vi "XYZ Table Stage Module.vi"(7 "Action":T4, 8 "Error In":errorcluster, 10 "Axis":enum16{"X Axis", "Y Axis", "Z Axis"}(ring), 11 "Control Param In":T2={"Position"=0.0, "Is.Enabled?"=FALSE, "Is.Connected?"=FALSE, "Device SN"="45876539", "AccelerationMaximum"=0.0, "VelocityMaximum"=0.0, "Acceleration"=0.0, "Velocity"=0.0, "waitTimeout (ms)"=0, "Model"=enum."None", "Is.Homed?"=FALSE}) -> (0 "Error Out":errorcluster)   [LabVIEW 2014]
uses:
  Controls/Translation Stage Cluster.ctl
  General/Controls/Translation Stage Types.ctl
  Controls/Motion Translation Module Control.ctl
  General/Controls/Set Get Controls.ctl
  HW Configurations.vi
  General/Controls/FGV Actions.ctl
panel:
  in  "Set/Get":T1=enum."Get"
  out "Control Param Out":T2={"Position"=0.0, "Is.Enabled?"=FALSE, "Is.Connected?"=FALSE, "Device SN"="45876539", "AccelerationMaximum"=0.0, "VelocityMaximum"=0.0, "Acceleration"=0.0, "Velocity"=0.0, "waitTimeout (ms)"=0, "Model"=enum."None", "Is.Homed?"=FALSE}
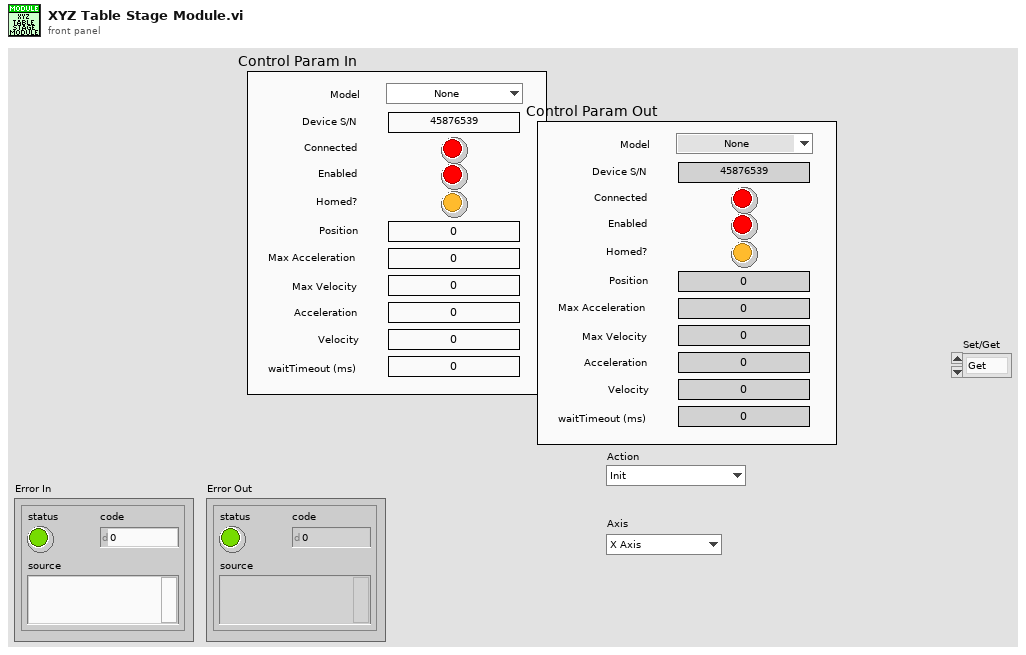
[diagram p1: front panel]
types:
  T1 = typedef "Set Get Controls.ctl" = enum16{"Set", "Get"}
  T2 = typedef "Translation Stage Cluster.ctl" = cluster{"Position":dbl, "Is.Enabled?":bool, "Is.Connected?":bool, "Device SN":string, "AccelerationMaximum":dbl, "VelocityMaximum":dbl, "Acceleration":dbl, "Velocity":dbl, "waitTimeout (ms)":i32, "Model":T3, "Is.Homed?":bool}
  T3 = typedef "Translation Stage Types.ctl" = enum16{"None", "Thorlabs LTS", "Thorlabs MLJ"}
  T4 = typedef "Motion Translation Module Control.ctl" = enum16{"Init", "Home", "Configure", "Velocity/Accel", "Position", "Jog", "Stop", "Uninit"}
  T5 = typedef "FGV Actions.ctl" = enum16{"Init", "Set", "Get", "Clear"}
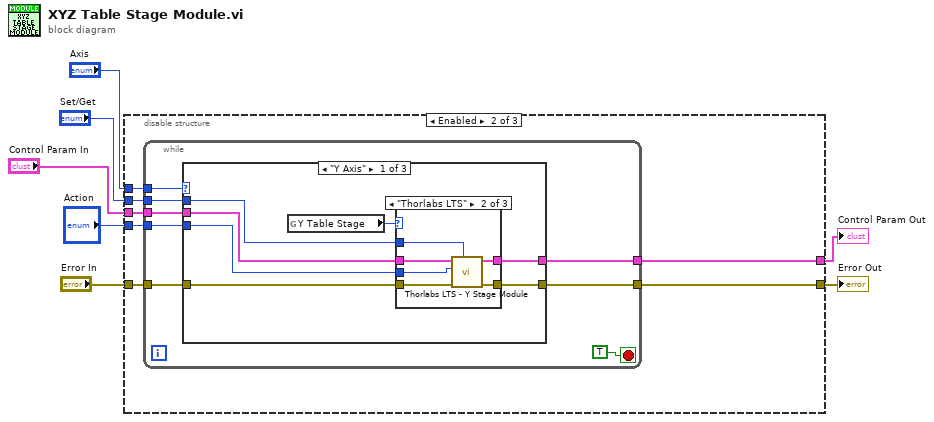
[diagram p0: block diagram]
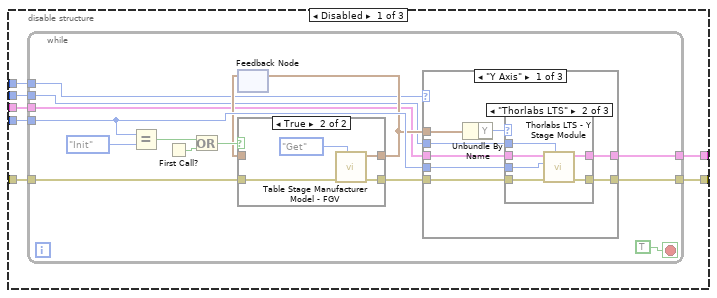
[diagram p2: hidden frame]
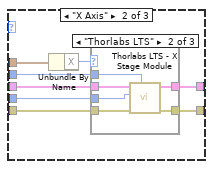
[diagram p5: hidden frame]
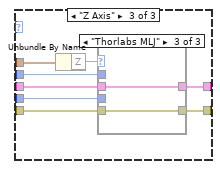
[diagram p8: hidden frame]
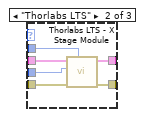
[diagram p10: hidden frame]
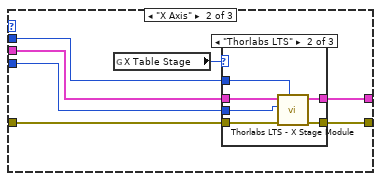
[diagram p14: hidden frame]
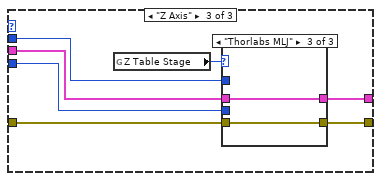
[diagram p17: hidden frame]
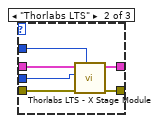
[diagram p19: hidden frame]
diagram:
  n1 = disable-structure shown="Enabled" {
    disable-tunnel: "Error In" -> [w14 w96 _]
    disable-tunnel: "Action" -> [w13 w95 _]
    disable-tunnel: [w12 w94 _] -> w5
    disable-tunnel: "Set/Get" -> [w11 w93 _]
    disable-tunnel: "Control Param In" -> [w10 w92 _]
    disable-tunnel: [w9 w91 _] -> w2
    disable-tunnel: "Axis" -> [w8 w90 _]
    frame Disabled {
      n2 = while {
        tunnel: w14 -> [w29]
        tunnel: w13 -> [w22]
        tunnel: [w21] -> w12
        tunnel: w11 -> [w18]
        tunnel: w10 -> [w17]
        tunnel: [w16] -> w9
        tunnel: w8 -> [w15]
        stop <- TRUE stop-if-true
        n3 = Equal?(x=w22, y=Motion_Translation_Module_Control."Init") -> (x = y?=w26:bool)
        n4 = First Call?() -> (First Call?: T/F=w27:bool)
        n5 = Or(x=w26, y=w27) -> (x .or. y?=w24:bool)
        n6 = feedback #1() -> (w19:cluster{"X":T3, "Y":T3, "Z":T3})  [unwired: 1 in]
        n7 = case shown="True" w24 {
          tunnel: [w85 w89] -> w23
          tunnel: w29 -> [w85 w88]
          tunnel: [w84 w86] -> w20
          tunnel: w19 -> [w84 _]
          frame False {
          }
          frame True {
            n8 = call "Table Stage Manufacturer Model - FGV.vi"("Actions"=FGV_Actions."Get", "Error In"=w88) -> ("Error Out"=w89:errorcluster, "Stage MFG/Model [Out]"=w86:cluster{"X":T3, "Y":T3, "Z":T3})  [unwired: 8 in]
          }
        }
        n9 = feedback-in #1(w20) -> ()
        n10 = case shown="\"Y Axis\"" w15 {
          tunnel: w23 -> [w37 w55 w73]
          tunnel: w22 -> [w36 w54 w72]
          tunnel: w20 -> [w35 w53 w71]
          tunnel: [w34 w52 w70] -> w21
          tunnel: w17 -> [w33 w51 w69]
          tunnel: [w32 w50 w68] -> w16
          tunnel: w18 -> [w30 w48 w66]
          frame "Y Axis" {
            n11 = Unbundle By Name(w35) -> ("Y"=w31:T3)
            n12 = case shown="\"Thorlabs LTS\"" w31 {
              tunnel: w37 -> [w39 w45 w47]
              tunnel: [w39 w44 w47] -> w34
              tunnel: w36 -> [_ w43 _]
              tunnel: w33 -> [w38 w42 w46]
              tunnel: [w38 w41 w46] -> w32
              tunnel: w30 -> [_ w40 _]
              frame "None", Default {
              }
              frame "Thorlabs LTS" {
                n13 = call "Thorlabs LTS - Y Stage Module.vi"("Set/Get"=w40, "Error In"=w45, "Action"=w43, "Cluster In"=w42) -> ("Error Out"=w44:errorcluster, "Cluster Out"=w41:T2)  [unwired: 6 in]
              }
              frame "Thorlabs MLJ" {
              }
            }
          }
          frame "X Axis" {
            n14 = Unbundle By Name(w53) -> ("X"=w49:T3)
            n15 = case shown="\"Thorlabs LTS\"" w49 {
              tunnel: w55 -> [w57 w63 w65]
              tunnel: [w57 w62 w65] -> w52
              tunnel: w54 -> [_ w59 _]
              tunnel: w51 -> [w56 w60 w64]
              tunnel: [w56 w61 w64] -> w50
              tunnel: w48 -> [_ w58 _]
              frame "None", Default {
              }
              frame "Thorlabs LTS" {
                n16 = call "Thorlabs LTS - X Stage Module.vi"("Set/Get"=w58, "Error In"=w63, "Action"=w59, "Cluster In"=w60) -> ("Error Out"=w62:errorcluster, "Cluster Out"=w61:T2)  [unwired: 6 in]
              }
              frame "Thorlabs MLJ" {
              }
            }
          }
          frame "Z Axis" {
            n17 = Unbundle By Name(w71) -> ("Z"=w67:T3)
            n18 = case shown="\"Thorlabs MLJ\"" w67 {
              tunnel: w73 -> [w75 w81 w83]
              tunnel: [w75 w80 w83] -> w70
              tunnel: w72 -> [_ w77 _]
              tunnel: w69 -> [w74 w78 w82]
              tunnel: [w74 w79 w82] -> w68
              tunnel: w66 -> [_ w76 _]
              frame "None", Default {
              }
              frame "Thorlabs LTS" {
                n19 = call "Thorlabs LTS - X Stage Module.vi"("Set/Get"=w76, "Error In"=w81, "Action"=w77, "Cluster In"=w78) -> ("Error Out"=w80:errorcluster, "Cluster Out"=w79:T2)  [unwired: 6 in]
              }
              frame "Thorlabs MLJ" {
              }
            }
          }
        }
      }
    }
    frame Enabled {
      n20 = while {
        tunnel: w96 -> [w97]
        tunnel: w95 -> [w103]
        tunnel: [w102] -> w94
        tunnel: w93 -> [w101]
        tunnel: w92 -> [w100]
        tunnel: [w99] -> w91
        tunnel: w90 -> [w98]
        stop <- TRUE stop-if-true
        n21 = case shown="\"Y Axis\"" w98 {
          tunnel: w97 -> [w111 w128 w145]
          tunnel: w103 -> [w110 w127 w144]
          tunnel: [w109 w126 w143] -> w102
          tunnel: w100 -> [w108 w125 w142]
          tunnel: [w107 w124 w141] -> w99
          tunnel: w101 -> [w106 w123 w140]
          frame "Y Axis" {
            n22 = global read "HW Configurations.vi" "Y Table Stage"() -> (w105:T3)
            n23 = case shown="\"Thorlabs LTS\"" w105 {
              tunnel: w111 -> [w113 w119 w121]
              tunnel: [w113 w118 w121] -> w109
              tunnel: w110 -> [_ w117 _]
              tunnel: w108 -> [w112 w116 w120]
              tunnel: [w112 w115 w120] -> w107
              tunnel: w106 -> [_ w114 _]
              frame "None", Default {
              }
              frame "Thorlabs LTS" {
                n24 = call "Thorlabs LTS - Y Stage Module.vi"("Set/Get"=w114, "Error In"=w119, "Action"=w117, "Cluster In"=w116) -> ("Error Out"=w118:errorcluster, "Cluster Out"=w115:T2)  [unwired: 6 in]
              }
              frame "Thorlabs MLJ" {
              }
            }
          }
          frame "X Axis" {
            n25 = global read "HW Configurations.vi" "X Table Stage"() -> (w122:T3)
            n26 = case shown="\"Thorlabs LTS\"" w122 {
              tunnel: w128 -> [w130 w136 w138]
              tunnel: [w130 w135 w138] -> w126
              tunnel: w127 -> [_ w132 _]
              tunnel: w125 -> [w129 w133 w137]
              tunnel: [w129 w134 w137] -> w124
              tunnel: w123 -> [_ w131 _]
              frame "None", Default {
              }
              frame "Thorlabs LTS" {
                n27 = call "Thorlabs LTS - X Stage Module.vi"("Set/Get"=w131, "Error In"=w136, "Action"=w132, "Cluster In"=w133) -> ("Error Out"=w135:errorcluster, "Cluster Out"=w134:T2)  [unwired: 6 in]
              }
              frame "Thorlabs MLJ" {
              }
            }
          }
          frame "Z Axis" {
            n28 = global read "HW Configurations.vi" "Z Table Stage"() -> (w139:T3)
            n29 = case shown="\"Thorlabs MLJ\"" w139 {
              tunnel: w145 -> [w147 w153 w155]
              tunnel: [w147 w152 w155] -> w143
              tunnel: w144 -> [_ w149 _]
              tunnel: w142 -> [w146 w150 w154]
              tunnel: [w146 w151 w154] -> w141
              tunnel: w140 -> [_ w148 _]
              frame "None", Default {
              }
              frame "Thorlabs LTS" {
                n30 = call "Thorlabs LTS - X Stage Module.vi"("Set/Get"=w148, "Error In"=w153, "Action"=w149, "Cluster In"=w150) -> ("Error Out"=w152:errorcluster, "Cluster Out"=w151:T2)  [unwired: 6 in]
              }
              frame "Thorlabs MLJ" {
              }
            }
          }
        }
      }
    }
    frame Disabled {
    }
  }
  "Error Out" <- w5
  "Control Param Out" <- w2
